vi "Start.vi"(7 "Alias Name":string, 8 "error in":errorcluster, 9 "Other Args":string, 10 "Port":i32, 11 "Micron Path":path) -> (0 "error out":errorcluster, 3 "Connection String":string)   [LabVIEW 2019, in "MicronClient.lvclass"]
uses:
  MicronClient.lvclass
  <vilib>/SLL Toolkit/SLL File IO/SLL File IO.lvlib
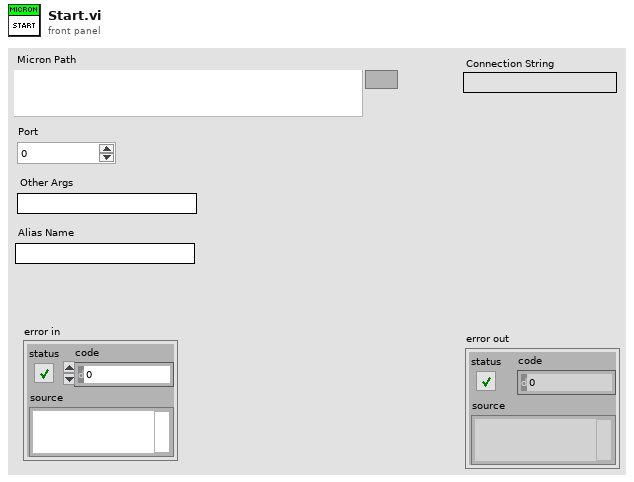
[diagram p1: front panel]
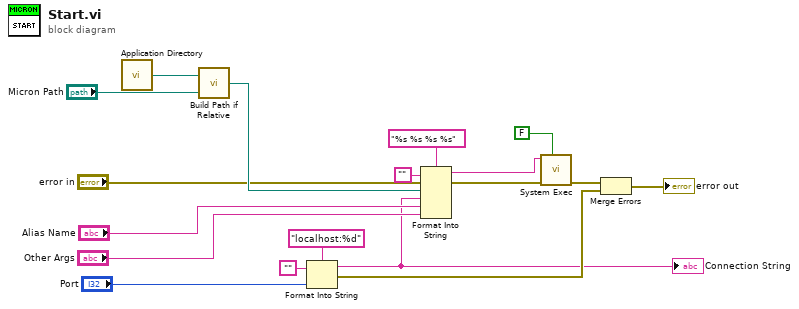
[diagram p0: block diagram]
diagram:
  n1 = call <vilib>:"Application Directory.vi"() -> ("Application Directory"=w13:path)
  n2 = call <vilib>:"Build Path if Relative.vi"("Relative or Absolute Path"="Micron Path", "Base Path"=w13) -> ("Path Out"=w12:path)
  n3 = Format Into String(format string="localhost:%d", initial string="", "Port") -> (resulting string=w1:string, error out=w2:errorcluster)  [unwired: 1 in]
  "Connection String" <- w1
  n4 = Format Into String(format string="%s %s %s %s", initial string="", error in="error in", w12, w1, "Alias Name", "Other Args") -> (resulting string=w14:string, error out=w17:errorcluster)
  n5 = call <vilib>:"System Exec.vi"("wait until completion? (T)"=FALSE, "error in (no error)"=w17, "command line"=w14) -> ("error out"=w7:errorcluster)  [unwired: 5 in, 3 out]
  n6 = Merge Errors(w7, w2) -> (→"error out":errorcluster)
